vi "Read to Queue.vi"   [LabVIEW 2014]
uses:
  Formula Hybrid 2012 r1/FPGA Telem for Slow Logging.ctl
  Formula Hybrid 2012 r1/Global Data.vi
types:
  T1 = cluster{"read mode":enum16{"polling", "blocking"}, "write mode":enum16{"polling", "blocking"}}
  T2 = typedef "FPGA Telem for Slow Logging.ctl" = cluster{"TSBRIO":fxp<+/-,16,9>, "VsbRIOSpply":fxp<+/-,25,6>, "bFPGALED":bool, "CPU Load":cluster{"Total (%)":dbl, "Time Critical (%)":dbl, "Timed Structures (%)":dbl, "High (%)":dbl, "Above Normal (%)":dbl, "Normal (%)":dbl, "Background (%)":dbl, "Idle (%)":dbl, "ISR (%)":dbl}, "Time Stamp":timestamp, "NLatiPhone":dbl, "NLongiPhone":dbl, "nGPSiPhone":dbl, "IHighCurrent":fxp<+/-,24,15>, "ILowCurrent":fxp<+/-,24,15>, "V5VSupply":fxp<+/-,24,5>, "tCurrentLap":u32, "tLastLap":u32, "NLap":u8, "bCoolantPumpEnable":bool, "bRTDSEnable":bool, "bTSMSInStatus":bool, "bPosAIREnable":bool, "bBMSOK":bool, "bIMDOK":bool, "bBSPDOK":bool, "bSBRIOOK2":bool, "bSBRIOOK1":bool, "bTSMSOutStatus":bool, "bMotorControllerEnable":bool, "Tire Diameter(m)":fxp<+,16,1>}
  T3 = cluster{"Total (%)":dbl, "Time Critical (%)":dbl, "Timed Structures (%)":dbl, "High (%)":dbl, "Above Normal (%)":dbl, "Normal (%)":dbl, "Background (%)":dbl, "Idle (%)":dbl, "ISR (%)":dbl}
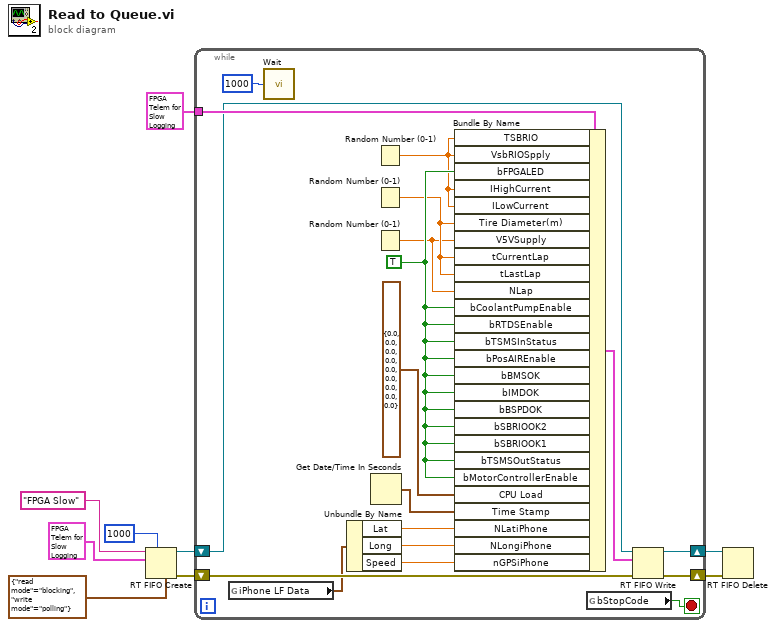
[diagram p0: block diagram]
diagram:
  n1 = RT FIFO Create(0:"FPGA Slow" ("name (unnamed)"), 1:T2 {"TSBRIO"=0.0, "VsbRIOSpply"=0.0, "bFPGALED"=FALSE, "CPU Load"={"Total (%)"=0.0, "Time Critical (%)"=0.0, "Timed Structures (%)"=0.0, "High (%)"=0.0, "Above Normal (%)"=0.0, "Normal (%)"=0.0, "Background (%)"=0.0, "Idle (%)"=0.0, "ISR (%)"=0.0}, "Time Stamp"=timestamp(0 s since 1904-01-01), "NLatiPhone"=0.0, "NLongiPhone"=0.0, "nGPSiPhone"=0.0, "IHighCurrent"=0.0, "ILowCurrent"=0.0, "V5VSupply"=-16.0, "tCurrentLap"=4, "tLastLap"=0, "NLap"=0, "bCoolantPumpEnable"=FALSE, "bRTDSEnable"=FALSE, "bTSMSInStatus"=FALSE, "bPosAIREnable"=FALSE, "bBMSOK"=TRUE, "bIMDOK"=TRUE, "bBSPDOK"=FALSE, "bSBRIOOK2"=FALSE, "bSBRIOOK1"=FALSE, "bTSMSOutStatus"=FALSE, "bMotorControllerEnable"=FALSE, "Tire Diameter(m)"=0.0} ("FPGA Logging Telem"), 4:u32 1000 ("size (10)"), 7:T1 {"read mode"=enum."blocking", "write mode"=enum."polling"} ("r/w modes (polling,polling)")) -> (8:w4:refnum<k33>, 11:w3:errorcluster)  [unwired: 4 in, 1 out]
  n2 = while {
    tunnel: T2 {"TSBRIO"=0.0, "VsbRIOSpply"=0.0, "bFPGALED"=FALSE, "CPU Load"={"Total (%)"=0.0, "Time Critical (%)"=0.0, "Timed Structures (%)"=0.0, "High (%)"=0.0, "Above Normal (%)"=0.0, "Normal (%)"=0.0, "Background (%)"=0.0, "Idle (%)"=0.0, "ISR (%)"=0.0}, "Time Stamp"=timestamp(0 s since 1904-01-01), "NLatiPhone"=0.0, "NLongiPhone"=0.0, "nGPSiPhone"=0.0, "IHighCurrent"=0.0, "ILowCurrent"=0.0, "V5VSupply"=-16.0, "tCurrentLap"=4, "tLastLap"=0, "NLap"=0, "bCoolantPumpEnable"=FALSE, "bRTDSEnable"=FALSE, "bTSMSInStatus"=FALSE, "bPosAIREnable"=FALSE, "bBMSOK"=TRUE, "bIMDOK"=TRUE, "bBSPDOK"=FALSE, "bSBRIOOK2"=FALSE, "bSBRIOOK1"=FALSE, "bTSMSOutStatus"=FALSE, "bMotorControllerEnable"=FALSE, "Tire Diameter(m)"=0.0} ("FPGA Logging Telem") -> [w27]
    shift-right: [w23] -> w1
    shift-left: w4 -> [w26]
    shift-right: [w22] -> w2
    shift-left: w3 -> [w25]
    stop <- w15 stop-if-true
    w13 = TRUE
    n3 = global read "Global Data.vi" "iPhone LF Data"() -> (w20:cluster{"Lat":dbl, "Long":dbl, "Speed":dbl})
    n4 = call "Wait"("Count(mSec)"=u32 1000) -> ()  [unwired: 1 out]
    n5 = Unbundle By Name(w20) -> ("Lat"=w18:dbl, "Long"=w17:dbl, "Speed"=w16:dbl)
    n6 = Get Date/Time In Seconds() -> (seconds since 1Jan1904=w19:timestamp)
    n7 = Random Number (0-1)() -> (number: 0 to 1=w12:dbl)
    n8 = Random Number (0-1)() -> (number: 0 to 1=w11:dbl)
    n9 = Random Number (0-1)() -> (number: 0 to 1=w10:dbl)
    n10 = Bundle By Name(cluster=w27, "TSBRIO"=w12, "VsbRIOSpply"=w12, "bFPGALED"=w13, "IHighCurrent"=w12, "ILowCurrent"=w12, "Tire Diameter(m)"=w11, "V5VSupply"=w10, "tCurrentLap"=w11, "tLastLap"=w11, "NLap"=w10, "bCoolantPumpEnable"=w13, "bRTDSEnable"=w13, "bTSMSInStatus"=w13, "bPosAIREnable"=w13, "bBMSOK"=w13, "bIMDOK"=w13, "bBSPDOK"=w13, "bSBRIOOK2"=w13, "bSBRIOOK1"=w13, "bTSMSOutStatus"=w13, "bMotorControllerEnable"=w13, "CPU Load"=T3 {"Total (%)"=0.0, "Time Critical (%)"=0.0, "Timed Structures (%)"=0.0, "High (%)"=0.0, "Above Normal (%)"=0.0, "Normal (%)"=0.0, "Background (%)"=0.0, "Idle (%)"=0.0, "ISR (%)"=0.0}, "Time Stamp"=w19, "NLatiPhone"=w18, "NLongiPhone"=w17, "nGPSiPhone"=w16) -> (w24:T2)
    n11 = global read "Global Data.vi" "bStopCode"() -> (w15:bool)
    n12 = RT FIFO Write(0:w26, 1:w24, 3:w25) -> (8:w23:refnum<k33>, 11:w22:errorcluster)  [unwired: 2 in, 2 out]
  }
  n13 = RT FIFO Delete(0:w1, 3:w2) -> ()  [unwired: 1 in, 1 out]
